vi "GLdrv_Write_TCPIP.vi"(0 "connection ID":refnum<k5>, 5 "data in":string, 11 "error in (no error)":errorcluster, 12 "timeout ms (25000)":i32) -> (4 "connection ID out":refnum<k5>, 15 "error out":errorcluster)   [LabVIEW 2017]
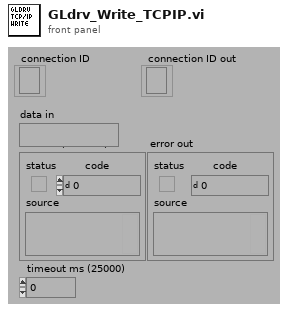
[diagram p1: front panel]
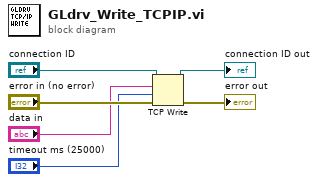
[diagram p0: block diagram]
diagram:
  n1 = TCP Write(connection ID="connection ID", data in="data in", error in (no error)="error in (no error)", 9:"timeout ms (25000)") -> (connection ID out=→"connection ID out":refnum<k5>, error out=→"error out":errorcluster)  [unwired: 1 out]
